vi "Progress Bar.vi"(6 "Multiple files?":bool) -> ()   [LabVIEW 2010]
uses:
  <vilib>/Utility/miscctls.llb/LVMinMaxIncTypeDef.ctl
  Progress.vi
panel:
  out "Processing multiple":u8(slide) max=100 step=1 scale=0.0..100.0
  out "Processing single":u8(slide) max=100 step=1 scale=0.0..100.0
  # "Processing"
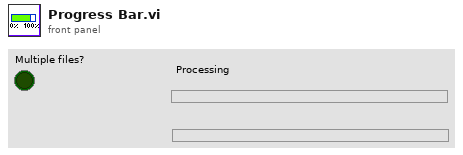
[diagram p1: front panel]
types:
  T1 = typedef "LVMinMaxIncTypeDef.ctl" = cluster{"Minimum":dbl, "Maximum":dbl, "Increment":dbl}
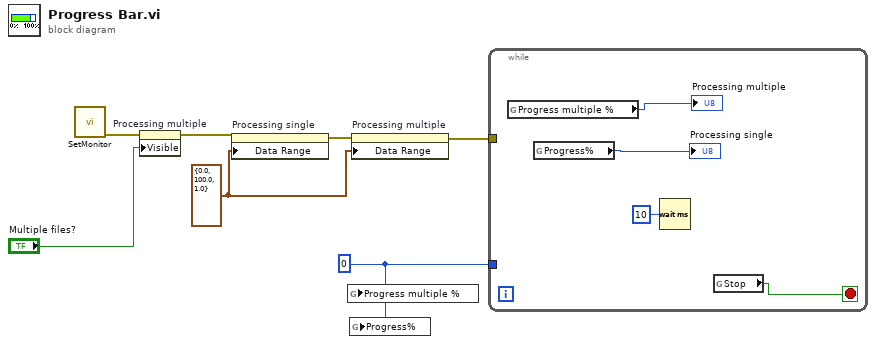
[diagram p0: block diagram]
diagram:
  w2 = u8 0 ("Generating")
  w6 = T1 {"Minimum"=0.0, "Maximum"=100.0, "Increment"=1.0} ("Min Max Inc")
  n1 = call "SetMonitor.vi"() -> ("error out"=w1:errorcluster)  [unwired: 10 in, 1 out]
  n2 = property on="Processing multiple" class="Slide (strict)"(error in=w1, "Visible"="Multiple files?") -> (error out=w4:errorcluster)  [unwired: 1 in, 1 out]
  n3 = property on="Processing single" class="Slide (strict)"(error in=w4, "Data Range"=w6) -> (error out=w5:errorcluster)  [unwired: 1 in, 1 out]
  n4 = global write "Progress.vi" "Progress multiple %"(w2) -> ()
  n5 = global write "Progress.vi" "Progress%"(w2) -> ()
  n6 = property on="Processing multiple" class="Slide (strict)"(error in=w5, "Data Range"=w6) -> (error out=w7:errorcluster)  [unwired: 1 in, 1 out]
  n7 = while {
    tunnel: w2 -> [_]
    tunnel: w7 -> [_]
    stop <- w10 stop-if-true
    n8 = global read "Progress.vi" "Progress multiple %"() -> (→"Processing multiple":u8)
    n9 = global read "Progress.vi" "Progress%"() -> (→"Processing single":u8)
    n10 = Wait (ms)(milliseconds to wait=u32 10) -> ()  [unwired: 1 out]
    n11 = global read "Progress.vi" "Stop"() -> (w10:bool)
  }
